vi "Injecting Report Class.vi"() -> ()   [LabVIEW 2009]
uses:
  classes/Test Suite/Test Suite.lvclass
  classes/Test Report.JUnit/Test Report.JUnit.lvclass
panel:
  in  "Report Path":path
  out "error out":errorcluster
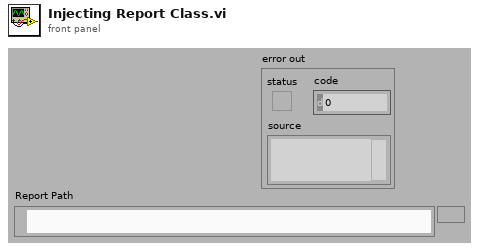
[diagram p1: front panel]
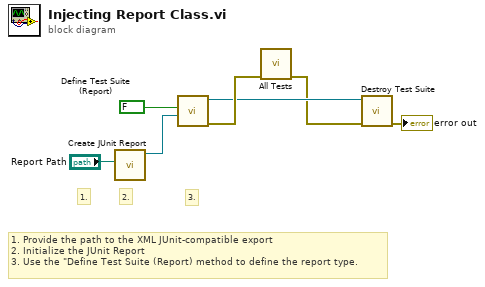
[diagram p0: block diagram]
diagram:
  # "3."
  # "2."
  # "1."
  # "1. Provide the path to the XML JUnit-compatible export\n2. Initialize the JUnit Report\n3. Use the \"Define Test Suite (Report) method to define the report type."
  n1 = call "Create JUnit Report.vi"("Report Path"="Report Path") -> ("Test Report.JUnit out"=w1:refnum<class "Test Report.JUnit.lvclass">)  [unwired: 9 in, 1 out]
  n2 = call "Define Test Suite (Report).vi"("Test Report"=w1, "Interactive"=FALSE) -> ("error out"=w7:errorcluster, "Test Suite"=w6:refnum<class "Test Suite.lvclass">)  [unwired: 8 in]
  n3 = call "All Tests.vi"("error in (no error)"=w7) -> ("error out"=w5:errorcluster)  [unwired: 10 in]
  n4 = call-dynamic "Destroy Test Suite.vi"("error in (no error)"=w5, "Test Suite in"=w6) -> ("error out"=→"error out":errorcluster)  [unwired: 9 in]
